vi "Signal_acquisition_v0.vi"() -> ()   [LabVIEW 2015]
uses:
  <vilib>/express/express analysis/Spectral/Block/exnSpectralBlock spectral measurements peak poly.vi
  <vilib>/express/express analysis/Spectral/Block/exnSpectralBlock spectral measurements peak WFM.vi
  <vilib>/measure/matone.llb/Extract Single Tone Information 1 Chan.vi
  <vilib>/express/express analysis/Spectral/XNode/ExpressSpectralMeasurementsBlockNode.xnode
  <vilib>/measure/NI_MAPro.lvlib
panel:
  out "Spectrum":cluster{"f0":dbl, "df":dbl, "magnitude":dbl[]}(graph)
  out "Frequency (MHz)":dbl
  out "Acquisition time complete":u32
  out "millisecond final timer":u32
  out "millisecond begin timer":u32
  out "millisecond timer value":u32
  out "detected frequency 2":dbl format="%.10f"
  out "detected frequency":dbl format="%.10f"
  in  "Channel #":u16(ring)=2 items=["Channel 1"=1, "Channel 2"=2]
  out "Numeric":i32
  out "data out":string
  in  "timeout ms (2000)":i32=2000
  in  "timeout ms (2000)":i32=2000
  in  "timeout ms (2000)":i32=2000
  in  "stop":bool
  out "error out":errorcluster
  out "Waveform Graph":dbl[](graph)
  in  "Trigger Mode":string(combo)="CH2_NE"
  in  "Pause for buffer (ms)":u32=100
  in  "Delay (# Samples)":i32 max=16348
  in  "Trigger Level (0 mV)":i32
  in  "IP address":string="192.168.1.139"
  in  "Decimation":u16(ring)=8 items=["65536"=65535, "8192"=8192, "1024"=1024, "64"=64, "8"=8, "1"=1]
  in  "error in":errorcluster
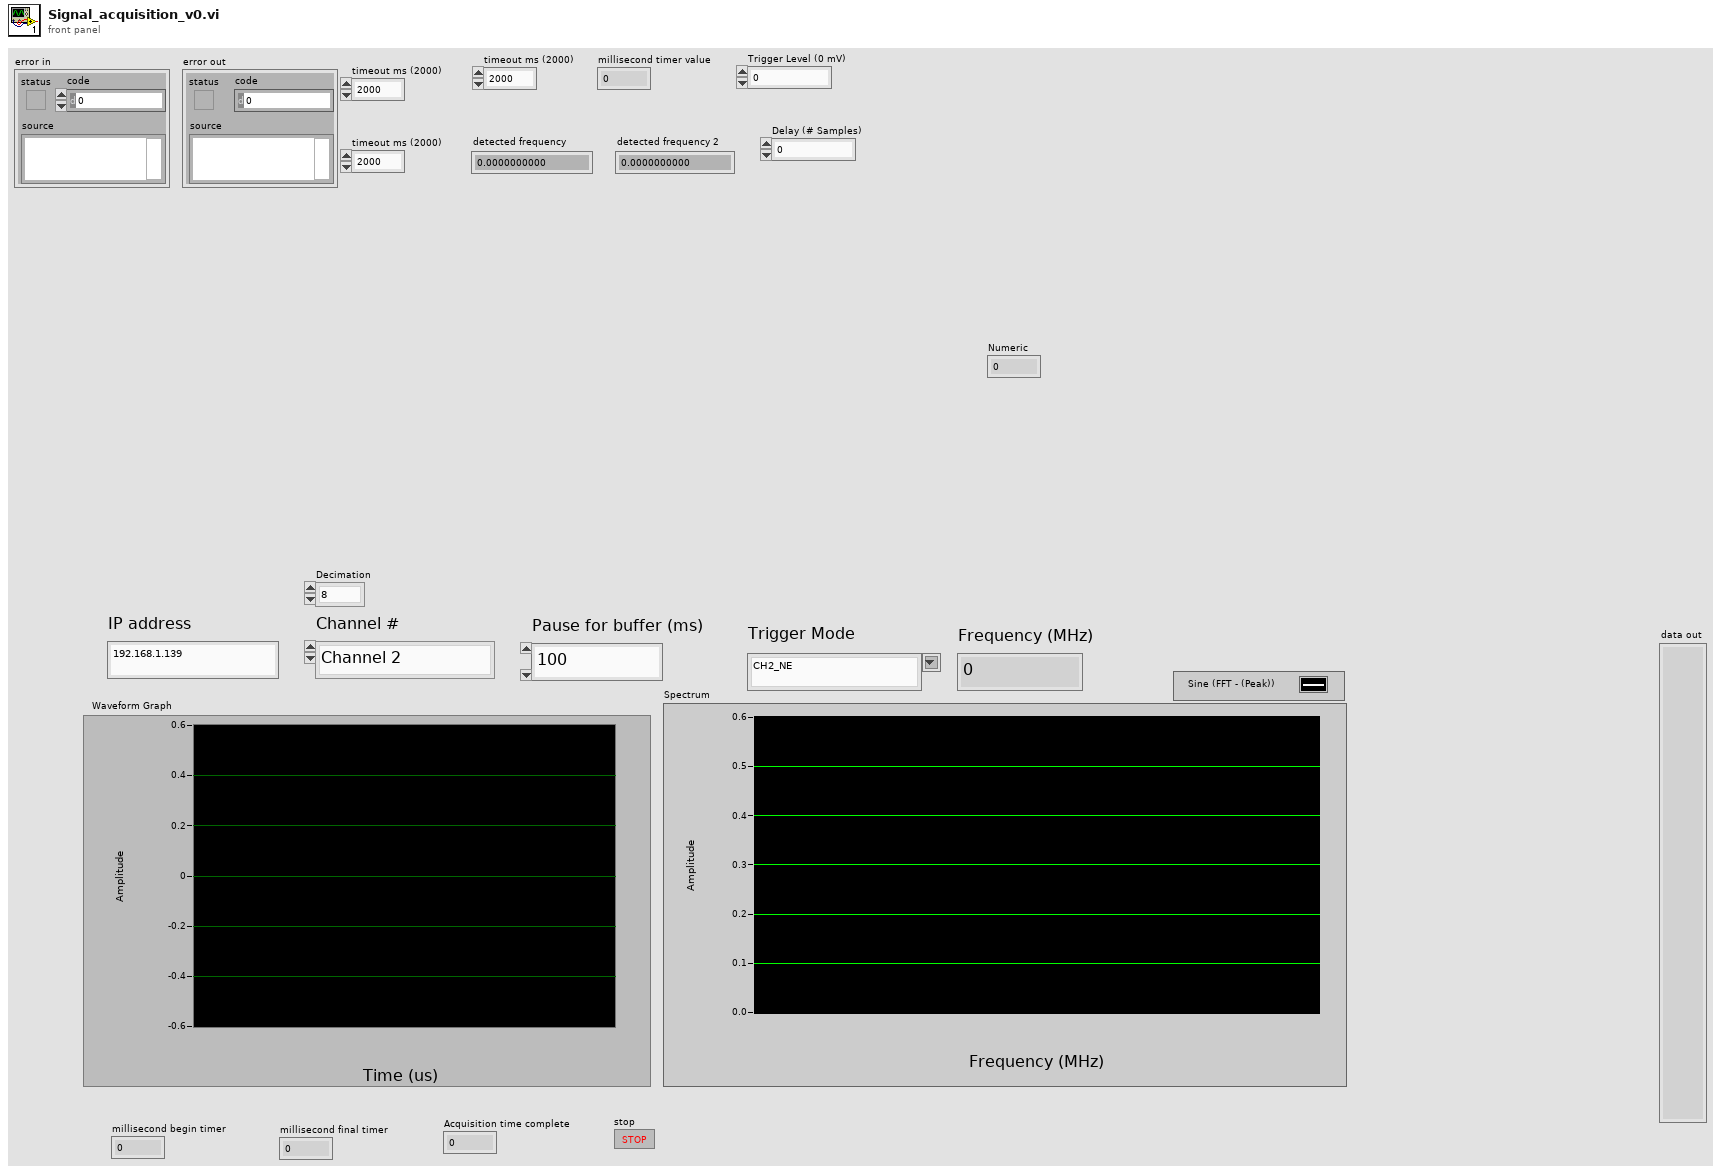
[diagram p1: front panel]
types:
  T1 = enum32{"none", "input signal", "detected signal", "residual signal"}
  T2 = enum16{"Standard", "Buffered", "CRLF", "Immediate"}
  T3 = cluster{"averaging mode":u16, "weighting mode":u16, "number of averages":u32}
  T4 = cluster{"dB On (F)":bool, "unwrap phase (F)":bool, "convert to degree (F)":bool}
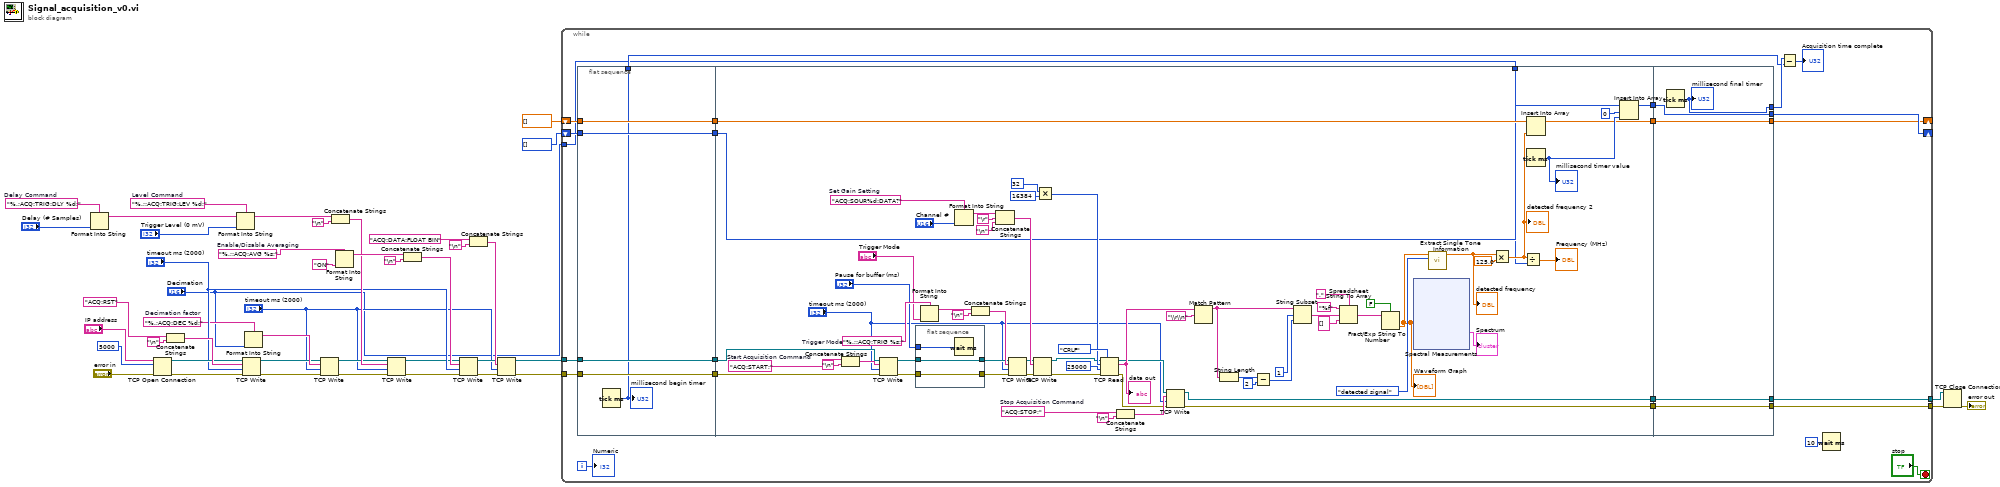
[diagram p0: block diagram]
diagram:
  w10 = "%.;:ACQ:AVG %s;"  # Enable/Disable Averaging
  w18 = "%.;ACQ:DEC %d;"  # Decimation factor
  w19 = "%.;ACQ:TRIG:DLY %d;"  # Delay Command
  w20 = "%.;:ACQ:TRIG:LEV %d;"  # Level Command
  n1 = Format Into String(format string=w19, "Delay (# Samples)") -> (resulting string=w38:string)  [unwired: 2 in, 1 out]
  n2 = TCP Open Connection(address="IP address", remote port or service name=u16 5000, error in (no error)="error in") -> (connection ID=w32:refnum<k5>, error out=w31:errorcluster)  [unwired: 2 in]
  n3 = Concatenate Strings("ACQ:RST" ("SCPI Message"), "\n") -> (w34:string)
  n4 = Format Into String(format string=w20, initial string=w38, "Trigger Level (0 mV)") -> (resulting string=w35:string)  [unwired: 1 in, 1 out]
  n5 = TCP Write(connection ID=w32, data in=w34, error in (no error)=w31, 9:"timeout ms (2000)") -> (connection ID out=w16:refnum<k5>, error out=w15:errorcluster)  [unwired: 1 out]
  n6 = Format Into String(format string=w18, "Decimation") -> (resulting string=w17:string)  [unwired: 2 in, 1 out]
  n7 = TCP Write(connection ID=w16, data in=w17, error in (no error)=w15, 9:"timeout ms (2000)") -> (connection ID out=w14:refnum<k5>, error out=w13:errorcluster)  [unwired: 1 out]
  n8 = Concatenate Strings(w35, "\n") -> (w29:string)
  n9 = Format Into String(format string=w10, "ON") -> (resulting string=w41:string)  [unwired: 2 in, 1 out]
  n10 = TCP Write(connection ID=w14, data in=w29, error in (no error)=w13, 9:"timeout ms (2000)") -> (connection ID out=w12:refnum<k5>, error out=w11:errorcluster)  [unwired: 1 out]
  n11 = Concatenate Strings(w41, "\n") -> (w30:string)
  n12 = TCP Write(connection ID=w12, data in=w30, error in (no error)=w11, 9:"timeout ms (2000)") -> (connection ID out=w8:refnum<k5>, error out=w7:errorcluster)  [unwired: 1 out]
  n13 = Concatenate Strings("ACQ:DATA:FLOAT BIN" ("SCPI Message"), "\n") -> (w26:string)
  n14 = TCP Write(connection ID=w8, data in=w26, error in (no error)=w7, 9:"timeout ms (2000)") -> (connection ID out=w5:refnum<k5>, error out=w4:errorcluster)  [unwired: 1 out]
  n15 = while {
    tunnel: w5 -> [w67]
    tunnel: [w59] -> w25
    tunnel: [w58] -> w24
    tunnel: w4 -> [w64]
    shift-right: [w63] -> _
    shift-left: u32[] [] -> [w61]
    shift-right: [w60] -> _
    shift-left: dbl[] [] -> [w62]
    tunnel: "Decimation" -> [w46]
    i -> [w65]
    stop <- "stop" stop-if-true
    n16 = flat-sequence {
      tunnel: w61 -> [w69]
      tunnel: w62 -> [w70]
      tunnel: w64 -> [w71]
      tunnel: w67 -> [w72]
      tunnel: [w72] -> w53
      tunnel: [w71] -> w52
      tunnel: [w70] -> w51
      tunnel: [w69] -> w50
      tunnel: [w68] -> w48
      tunnel: [w90] -> w57
      tunnel: [w87] -> w56
      tunnel: [w85] -> w55
      tunnel: [w80] -> w54
      tunnel: w53 -> [w134]
      tunnel: w52 -> [w97]
      tunnel: w51 -> [w89]
      tunnel: w50 -> [w88]
      tunnel: w46 -> [w75]
      tunnel: [w152] -> w58
      tunnel: [w153] -> w59
      tunnel: [w154] -> w60
      tunnel: [w155] -> w63
      tunnel: w57 -> [w155]
      tunnel: w56 -> [w154]
      tunnel: w55 -> [w153]
      tunnel: w54 -> [w152]
      tunnel: [w151] -> w49
      frame #0 {
        n17 = Tick Count (ms)() -> (millisecond timer value=w68:u32)
        "millisecond begin timer" <- w68
      }
      frame #1 {
        w84 = "ACQ:STOP;"  # Stop Acquisition Command
        w106 = "ACQ:SOUR%d:DATA?"  # Set Gain Setting
        w133 = "%.;:ACQ:TRIG %s;"  # Trigger Mode
        w136 = "ACQ:START;"  # Start Acquisition Command
        n18 = Concatenate Strings(w136, "\n") -> (w137:string)
        n19 = TCP Write(connection ID=w134, data in=w137, error in (no error)=w97, 9:"timeout ms (2000)") -> (connection ID out=w110:refnum<k5>, error out=w109:errorcluster)  [unwired: 1 out]
        n20 = flat-sequence {
          tunnel: "Pause for buffer (ms)" -> [w150]
          tunnel: [w149] -> w108
          tunnel: [w148] -> w107
          tunnel: w110 -> [w149]
          tunnel: w109 -> [w148]
          frame #0 {
            n21 = Wait (ms)(milliseconds to wait=w150) -> ()  [unwired: 1 out]
          }
        }
        n22 = Format Into String(format string=w133, "Trigger Mode") -> (resulting string=w130:string)  [unwired: 2 in, 1 out]
        n23 = Format Into String(format string=w106, "Channel #") -> (resulting string=w103:string)  [unwired: 2 in, 1 out]
        n24 = Concatenate Strings(w130, "\n") -> (w131:string)
        n25 = Concatenate Strings(w103, "\r", "\n") -> (w102:string)
        n26 = TCP Write(connection ID=w108, data in=w131, error in (no error)=w107, 9:"timeout ms (2000)") -> (connection ID out=w100:refnum<k5>, error out=w99:errorcluster)  [unwired: 1 out]
        n27 = TCP Write(connection ID=w100, data in=w102, error in (no error)=w99) -> (connection ID out=w101:refnum<k5>, error out=w98:errorcluster)  [unwired: 1 in, 1 out]
        n28 = Multiply(x=32, y=16384 ("bytes to read")) -> (x*y=w111:i32)
        n29 = TCP Read(connection ID=w101, bytes to read=w111, error in (no error)=w98, 7:T2."CRLF" ("mode (standard)"), 9:25000 ("timeout ms (25000)")) -> (connection ID out=w86:refnum<k5>, data out=w112:string, error out=w81:errorcluster)
        "data out" <- w112
        n30 = Concatenate Strings(w84, "\n") -> (w82:string)
        n31 = TCP Write(connection ID=w86, data in=w82, error in (no error)=w81, 9:"timeout ms (2000)") -> (connection ID out=w85:refnum<k5>, error out=w80:errorcluster)  [unwired: 1 out]
        n32 = Match Pattern(string=w112, regular expression="\\r\\n") -> (before substring=w118:string)  [unwired: 1 in, 3 out]
        n33 = String Length(string=w118) -> (length=w121:i32)
        n34 = Subtract(x=w121, y=2) -> (x-y=w122:i32)
        n35 = String Subset(string=w118, offset (0)=1, length (rest)=w122) -> (substring=w119:string)
        n36 = Spreadsheet String To Array(delimiter (Tab)=",", format string="%f", spreadsheet string=w119, array type (2D Dbl)=string[] [] ("Array")) -> (array=w125:string[])
        n37 = Fract/Exp String To Number(use system decimal point (T)=FALSE, string=w125) -> (number=w73:dbl[])  [unwired: 3 out]
        "Waveform Graph" <- w73
        n38 = xnode "Spectral Measurements"("Signals"=w73) -> ("FFT - (Peak)"=→"Spectrum":cluster{"f0":dbl, "df":dbl, "magnitude":dbl[]})  [unwired: 1 in, 2 out]
        n39 = call-poly <vilib>:"Extract Single Tone Information.vi"("export mode"=T1."detected signal", "time signal in"=w73) -> ("detected frequency"=w94:dbl)  [unwired: 4 in, 5 out]
        "detected frequency" <- w94
        n40 = Multiply(x=w94, y=125.0) -> (x*y=w76:dbl)
        "detected frequency 2" <- w76
        n41 = Divide(x=w76, y=w75) -> (x/y=→"Frequency (MHz)":dbl)
        n42 = Insert Into Array(array=w89, new element=w76) -> (w87:dbl[])  [unwired: 1 in]
        n43 = Tick Count (ms)() -> (millisecond timer value=w91:u32)
        "millisecond timer value" <- w91
        n44 = Insert Into Array(array=w88, index=0, new element=w91) -> (w90:u32[])
      }
      frame #2 {
        n45 = Tick Count (ms)() -> (millisecond timer value=w151:u32)
        "millisecond final timer" <- w151
      }
    }
    n46 = Subtract(x=w49, y=w48) -> (x-y=→"Acquisition time complete":u32)
    n47 = Wait (ms)(milliseconds to wait=u32 10) -> ()  [unwired: 1 out]
    "Numeric" <- w65
  }
  n48 = TCP Close Connection(connection ID=w25, error in (no error)=w24) -> (error out=→"error out":errorcluster)  [unwired: 1 in, 1 out]
